vi "open.vi"(0 "3_amp_volt in":refnum<class "3_amp_volt.lvclass">, 2 "Slave ID":u8=1, 3 "error in (no error)":errorcluster) -> (7 "3_amp_volt out":refnum<class "3_amp_volt.lvclass">, 10 "error out":errorcluster)   [LabVIEW 2018, in "3_amp_volt.lvclass"]
uses:
  3_amp_volt.lvclass
  3_amp_volt.lvclass/3_amp_volt.ctl
  <vilib>/Plasmionique/MB Master/MB_Master_Serial/MB_Master_Serial.lvclass
panel:
  in  "Serial Config":T1={"baud rate (bps)"=9600, "stop bits"=10, "parity"=0, "flow control"=0, "timeout"=1000, "retries"=1} {"stop bits" items=["1.0"=10, "1.5"=15, "2.0"=20]; "flow control" items=["None", "XON/XOFF", "RTS/CTS", "XON/XOFF & RTS/CTS", "DTR/DSR", "XON/XOFF & DTR/DSR"]; "parity" items=["None", "Odd", "Even", "Mark", "Space"]}
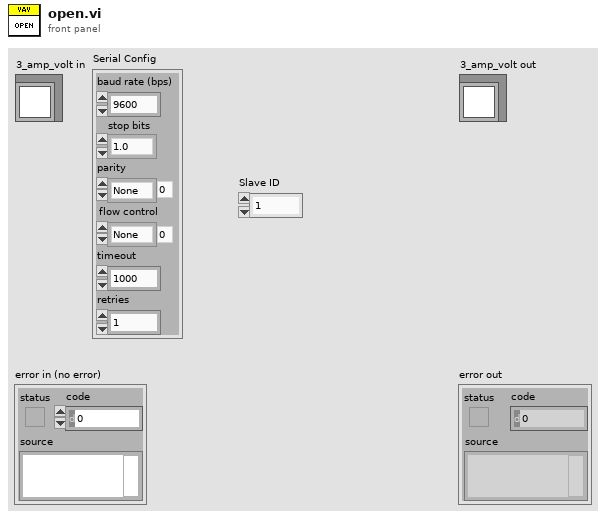
[diagram p1: front panel]
types:
  T1 = cluster{"baud rate (bps)":u32, "stop bits":u16, "parity":u16, "flow control":u16, "timeout":u32, "retries":i32}
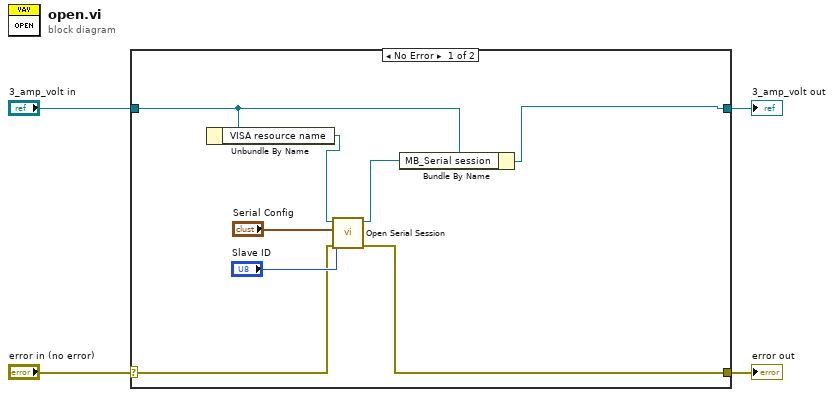
[diagram p0: block diagram]
diagram:
  n1 = case shown="No Error" "error in (no error)" {
    selector: "error in (no error)" -> [w9 w14]
    tunnel: [w8 w14] -> w3
    tunnel: [w5 w13] -> w1
    tunnel: "3_amp_volt in" -> [w6 w13]
    frame No Error {
      n2 = Unbundle By Name(w6) -> ("VISA resource name"=w10:refnum<visa-resource-name>)
      n3 = call <vilib>:"Open Serial Session.vi"("Error in"=w9, "Slave ID"="Slave ID", "Serial Config"="Serial Config", "VISA Resource"=w10) -> ("Error out"=w8:errorcluster, "MB_Serial session"=w7:refnum<class "MB_Master_Serial.lvclass">)  [unwired: 6 in]
      n4 = Bundle By Name(cluster=w6, "MB_Serial session"=w7) -> (w5:refnum<class "3_amp_volt.lvclass">)
    }
    frame Error {
    }
  }
  "error out" <- w3
  "3_amp_volt out" <- w1
